vi "test!!!!!!.vi"() -> ()   [LabVIEW 2019]
panel:
  out "sce-pannel-list out 2":T1(array[cluster]) {"pannel"."ID" format="%02x"}
  in  "停止":bool
  out "sce-pannel-list 2":T2(array[cluster])
  out "输出簇":cluster{"字符串":string, "数组 2":string[]}
  out "元素":T3
  out "sce-pannel-list out":T1(array[cluster]) {"pannel"."ID" format="%02x"}
  in  "索引":i32
  in  "模式列表 5":T4(array[cluster])=[{"模式"="关|睡眠模式", "sce-pannel-list"=[{"pannel"=[{"ID"=1, "type"="dev", "flag"="", "name"="第三方", "Act"={"Attribute"="", "Action"="open", "Value"=0.0}}, {"ID"=2, "type"="dev", "flag"="", "name"="水电费", "Act"={"Attribute"="", "Action"="close", "Value"=0.0}}, {"ID"=3, "type"="dev", "flag"="", "name"="二", "Act"={"Attribute"="", "Action"="open", "Value"=0.0}}], "pannel-id"=1.0}, {"pannel"=[{"ID"=1, "type"="dev", "flag"="", "name"="而风蛋糕", "Act"={"Attribute"="", "Action"="open", "Value"=0.0}}, {"ID"=2, "type"="dev", "flag"="", "name"="官方", "Act"={"Attribute"="", "Action"="open", "Value"=0.0}}, {"ID"=3, "type"="dev", "flag"="", "name"="俄文", "Act"={"Attribute"="", "Action"="close", "Value"=0.0}}], "pannel-id"=2.0}]}, {"模式"="开|睡眠模式", "sce-pannel-list"=[{"pannel"=[{"ID"=1, "type"="dev", "flag"="", "name"="而风蛋糕", "Act"={"Attribute"="", "Action"="open", "Value"=0.0}}, {"ID"=2, "type"="dev", "flag"="", "name"="官方", "Act"={"Attribute"="", "Action"="open", "Value"=0.0}}, {"ID"=3, "type"="dev", "flag"="", "name"="俄文", "Act"={"Attribute"="", "Action"="close", "Value"=0.0}}], "pannel-id"=2.0}]}, {"模式"="起床模式", "sce-pannel-list"=[{"pannel"=[{"ID"=1, "type"="dev", "flag"="", "name"="而风蛋糕", "Act"={"Attribute"="", "Action"="open", "Value"=0.0}}, {"ID"=2, "type"="dev", "flag"="", "name"="官方", "Act"={"Attribute"="", "Action"="open", "Value"=0.0}}, {"ID"=3, "type"="dev", "flag"="", "name"="俄文", "Act"={"Attribute"="", "Action"="close", "Value"=0.0}}], "pannel-id"=2.0}]}] {"sce-pannel-list"."pannel"."ID" format="%02x"}
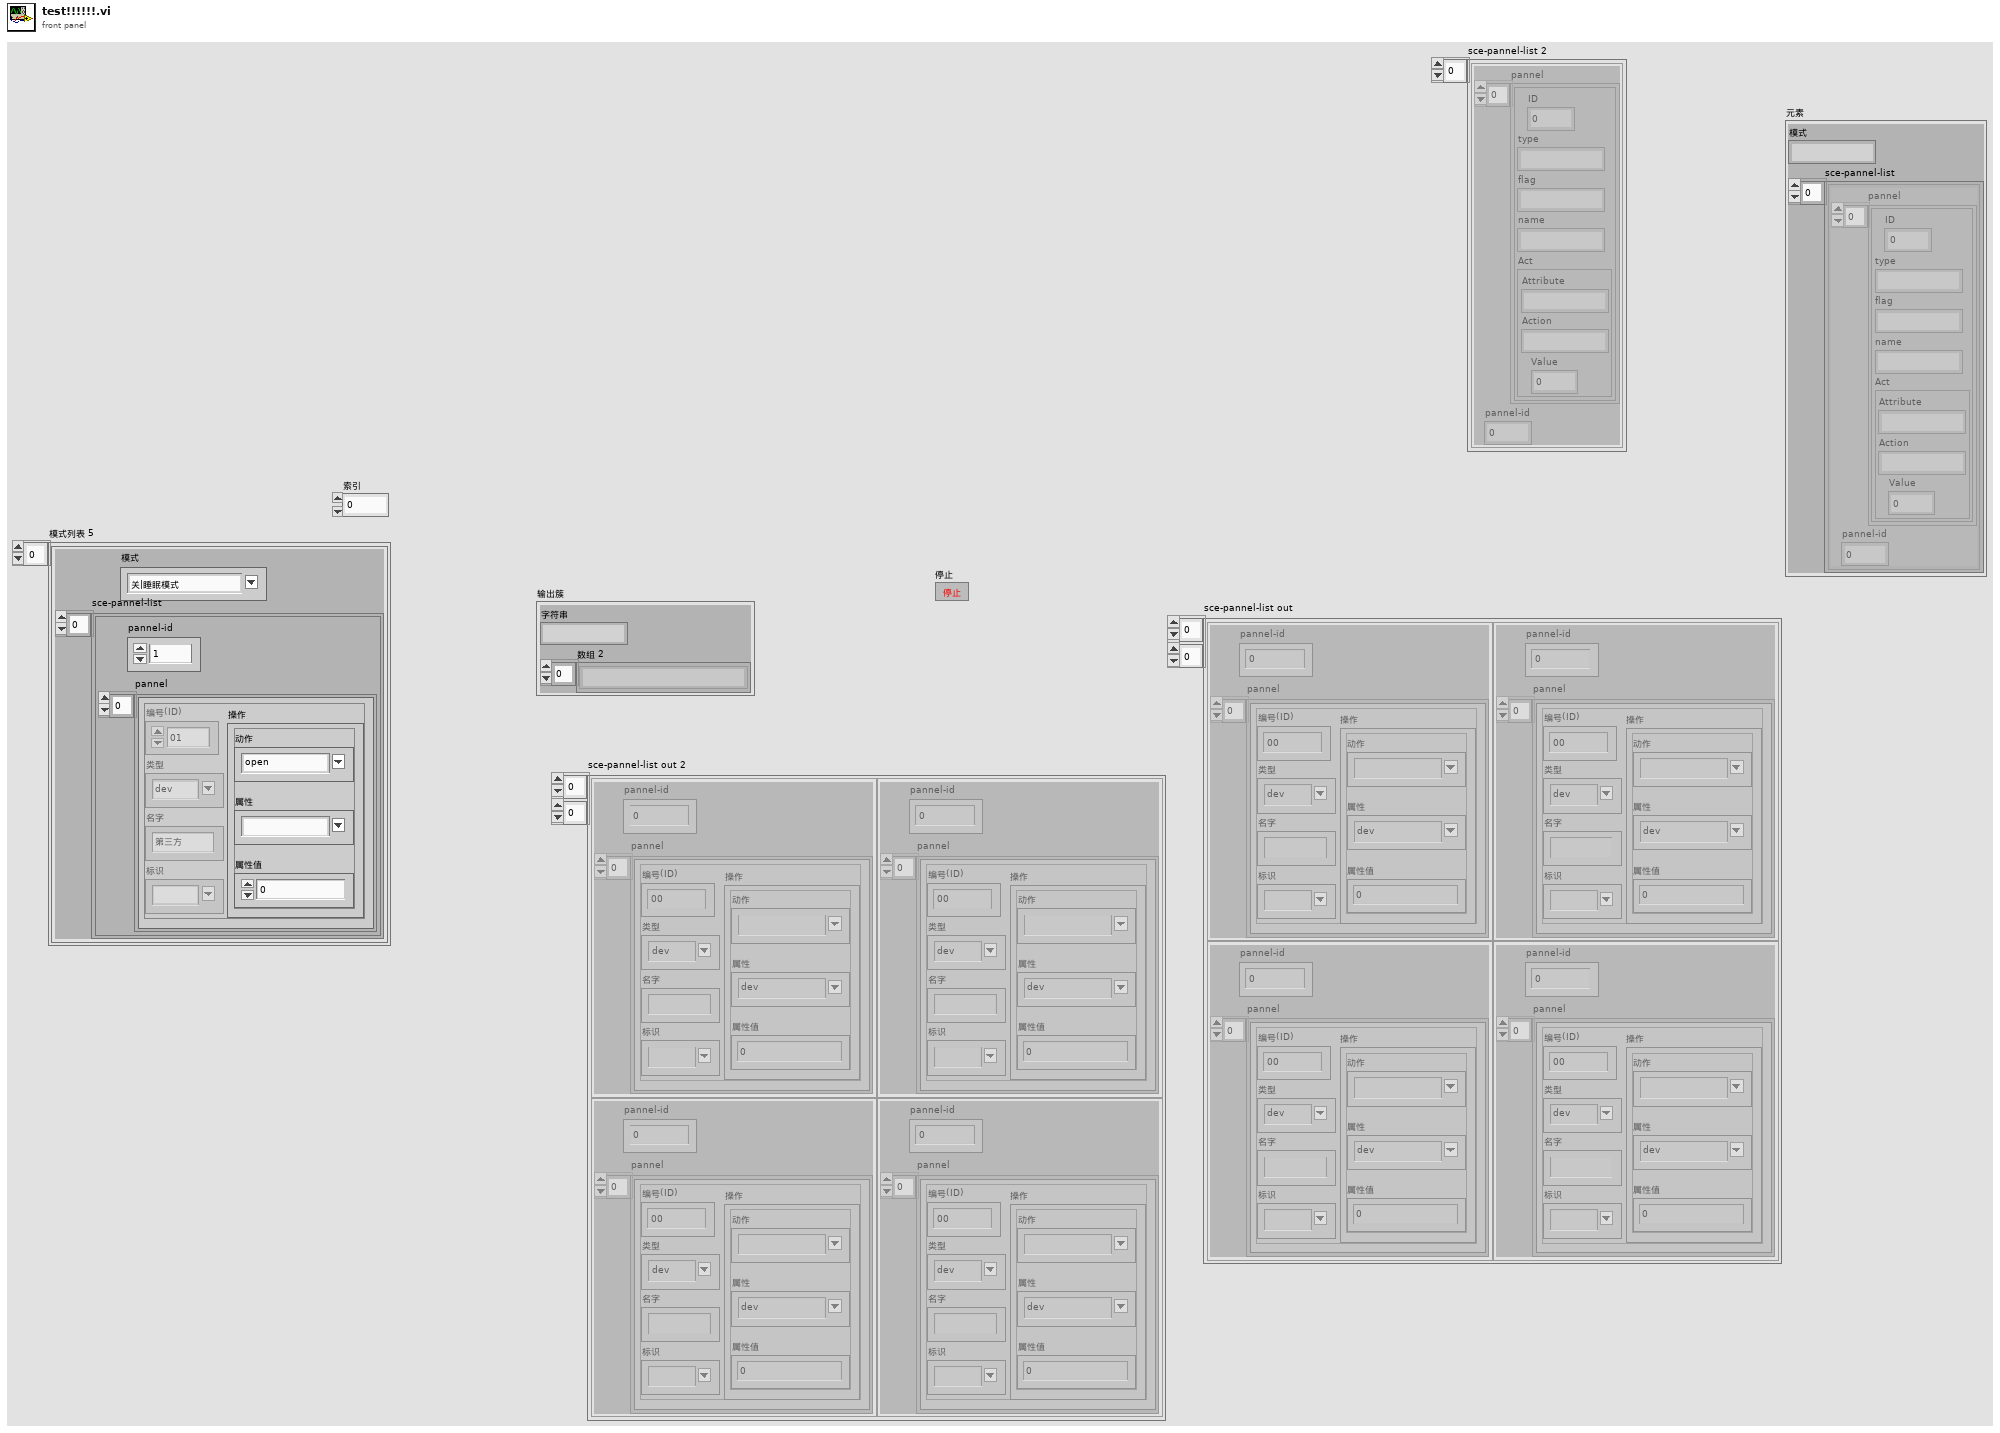
[diagram p1: front panel]
types:
  T1 = cluster{"pannel":cluster{"ID":u8, "type":string, "flag":string, "name":string, "Act":cluster{"Attribute":string, "Action":string, "Value":dbl}}[], "pannel-id":dbl}[][]
  T2 = cluster{"pannel":cluster{"ID":u8, "type":string, "flag":string, "name":string, "Act":cluster{"Attribute":string, "Action":string, "Value":dbl}}[], "pannel-id":dbl}[]
  T3 = cluster{"模式":string, "sce-pannel-list":cluster{"pannel":cluster{"ID":u8, "type":string, "flag":string, "name":string, "Act":cluster{"Attribute":string, "Action":string, "Value":dbl}}[], "pannel-id":dbl}[]}
  T4 = cluster{"模式":string, "sce-pannel-list":cluster{"pannel":cluster{"ID":u8, "type":string, "flag":string, "name":string, "Act":cluster{"Attribute":string, "Action":string, "Value":dbl}}[], "pannel-id":dbl}[]}[]
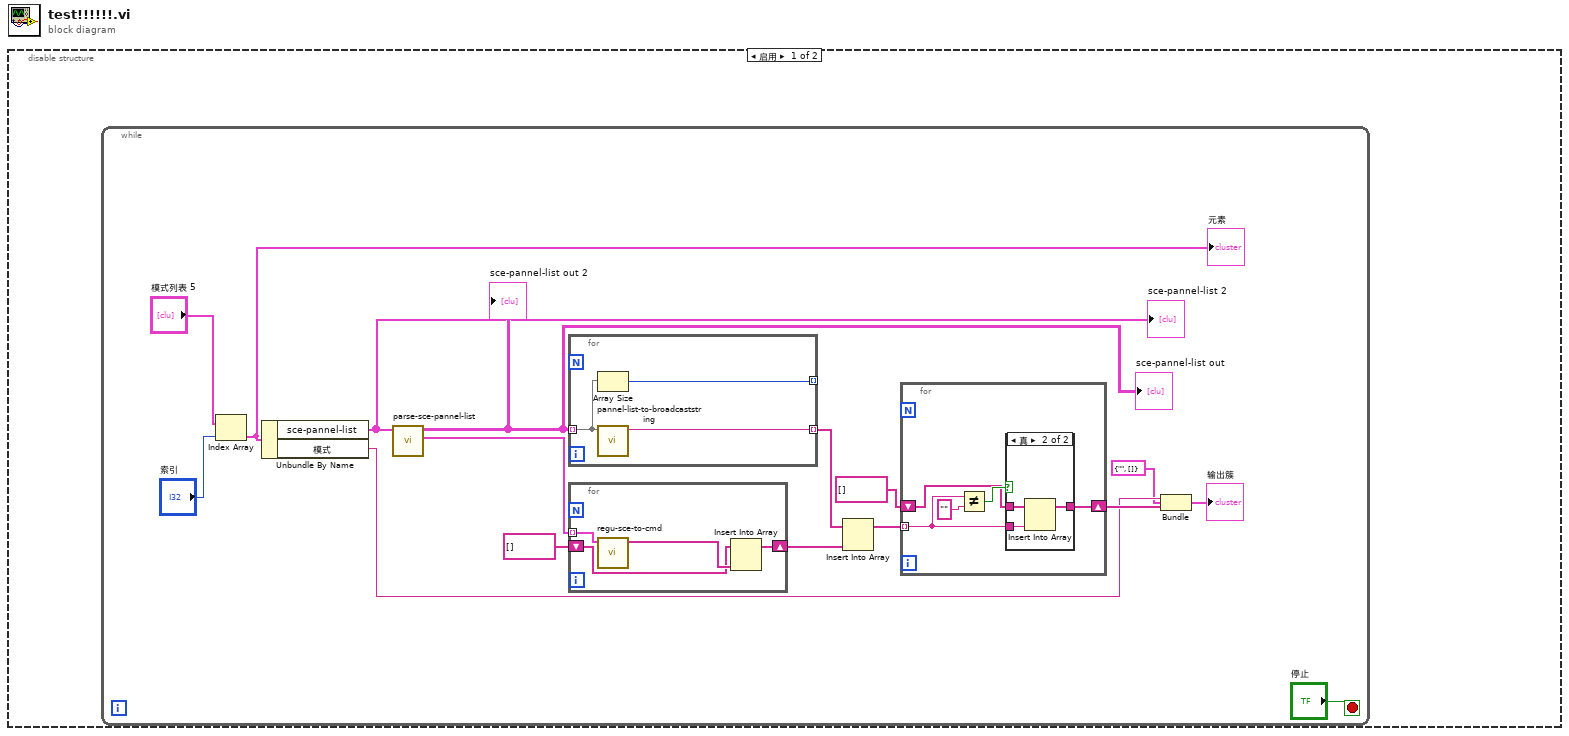
[diagram p0: block diagram]
diagram:
  n1 = disable-structure shown="启用" {
    frame Enabled {
      n2 = while {
        stop <- "停止" stop-if-true
        n3 = Index Array(array="模式列表 5", index="索引") -> (element=w5:T3)
        "元素" <- w5
        n4 = Unbundle By Name(w5) -> ("sce-pannel-list"=w6:T2, "模式"=w8:string)
        "sce-pannel-list 2" <- w6
        n5 = call "parse-sce-pannel-list.vi"("sce-pannel-list"=w6) -> ("sce-regulate-list"=w9:T2, "sce-pannel-list out"=w16:T1)  [unwired: 9 in]
        "sce-pannel-list out" <- w16
        "sce-pannel-list out 2" <- w16
        n6 = for {
          tunnel: w16 -> [w31] mode=indexing
          tunnel: [w32] -> w10 mode=indexing
          tunnel: [w30] -> _ mode=indexing
          n7 = Array Size(array=w31) -> (size(s)=w30:i32)
          n8 = call "pannel-list-to-broadcaststring.vi"("sce-pannel-list"=w31) -> ("sce-pannel-list-cmd"=w32:string)  [unwired: 10 in]
        }
        n9 = for {
          tunnel: w9 -> [w29] mode=indexing
          shift-right: [w27] -> w12
          shift-left: string[] [] -> [w26]
          n10 = call "regu-sce-to-cmd.vi"("regulate-pannel"=w29) -> ("regulate-cmd"=w28:string[])  [unwired: 10 in]
          n11 = Insert Into Array(array=w26, new element=w28) -> (w27:string[])  [unwired: 1 in]
        }
        n12 = Insert Into Array(array=w10, new element=w12) -> (w14:string[])  [unwired: 1 in]
        n13 = for {
          tunnel: w14 -> [w19] mode=indexing
          shift-right: [w18] -> w15
          shift-left: string[] [] -> [w17]
          n14 = Not Equal?(x=w19, y="") -> (x != y?=w20:bool)
          n15 = case shown="真" w20 {
            tunnel: w19 -> [_ w25]
            tunnel: [w22 w24] -> w18
            tunnel: w17 -> [w22 w23]
            frame False {
            }
            frame True {
              n16 = Insert Into Array(array=w23, new element=w25) -> (w24:string[])  [unwired: 1 in]
            }
          }
        }
        n17 = Bundle(cluster=cluster{"字符串":string, "数组 2":string[]} {"字符串"="", "数组 2"=[]} ("簇"), "字符串"=w8, "数组 2"=w15) -> (→"输出簇":cluster{"字符串":string, "数组 2":string[]})
      }
    }
    frame Disabled {
    }
  }
